vi "adam-check-DO-reply.vi"(8 "error in (no error)":errorcluster, 9 "Desired State":bool, 11 "VISA Refnum in":refnum<visa-resource-name>) -> (0 "error out":errorcluster, 2 "Channel Active":bool, 3 "VISA Refnum out":refnum<visa-resource-name>, 4 "read buffer":string, 5 "Status":string)   [LabVIEW 2024]
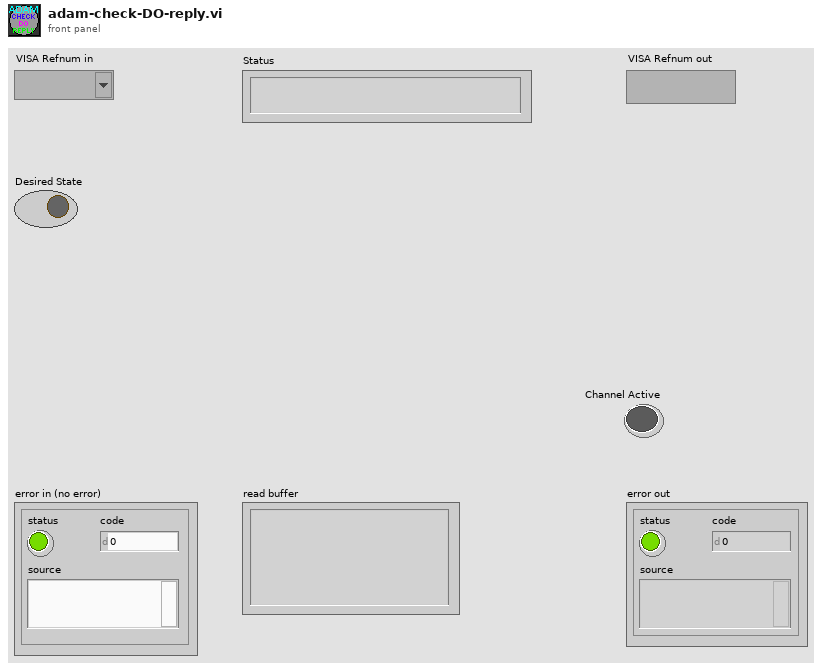
[diagram p1: front panel]
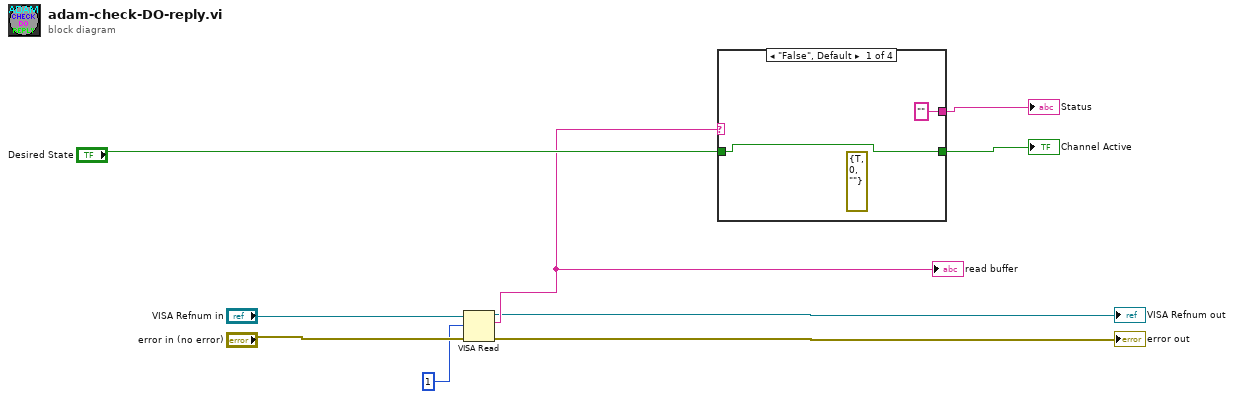
[diagram p0: block diagram]
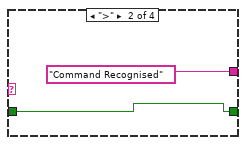
[diagram p2: hidden frame]
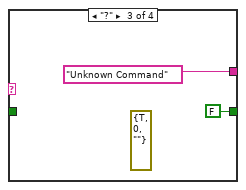
[diagram p3: hidden frame]
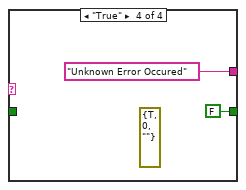
[diagram p4: hidden frame]
diagram:
  n1 = VISA Read(VISA resource name="VISA Refnum in", byte count=u32 1, error in (no error)="error in (no error)") -> (VISA resource name out=→"VISA Refnum out":refnum<visa-resource-name>, read buffer=w6:string, error out=→"error out":errorcluster)  [unwired: 1 out]
  "read buffer" <- w6
  n2 = case shown="\"False\", Default" w6 {
    tunnel: ["" ("Status") "Command Recognised" ("Status") "Unknown Command" ("Status") "Unknown Error Occured" ("Status")] -> w7
    tunnel: [w10 w12 FALSE FALSE] -> w8
    tunnel: "Desired State" -> [w10 w12 _ _]
    frame "False", Default {
      (unwired) errorcluster {"status"=TRUE, "code"=0, "source"=""} ("error in")
    }
    frame ">" {
    }
    frame "?" {
      (unwired) errorcluster {"status"=TRUE, "code"=0, "source"=""} ("error in")
    }
    frame "True" {
      (unwired) errorcluster {"status"=TRUE, "code"=0, "source"=""} ("error in")
    }
  }
  "Channel Active" <- w8
  "Status" <- w7
